vi "_wrapEditPosition.vi"(4 "TreeRef":refnum<vi>) -> (1 "Edit Position":cluster{"Row":i32, "Column":i32})   [LabVIEW 2017]
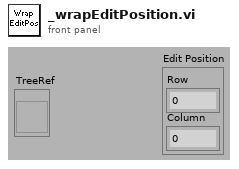
[diagram p1: front panel]
types:
  T1 = typedef "LVRowAndColumnTypeDef.ctl" = cluster{"Row":i32, "Column":i32}
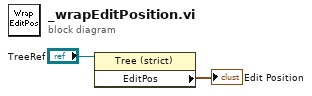
[diagram p0: block diagram]
diagram:
  n1 = property class="Tree (strict)"(reference="TreeRef") -> ("EditPos"=→"Edit Position":T1)  [unwired: 1 in, 2 out]
